vi "Valid.vi"(11 "ObserverSet in":refnum<class "ObserverSet.lvclass">) -> (2 "Valid?":bool, 3 "ObserverSet out":refnum<class "ObserverSet.lvclass">)   [LabVIEW 2011, in "Messenging.lvlib" / "ObserverSet.lvclass"]
uses:
  ObserverSet.lvclass
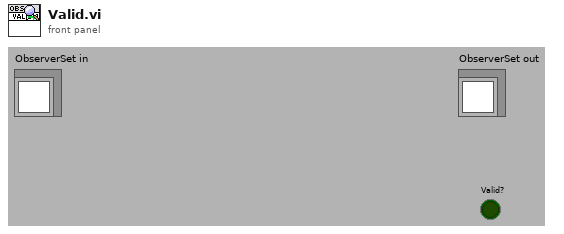
[diagram p1: front panel]
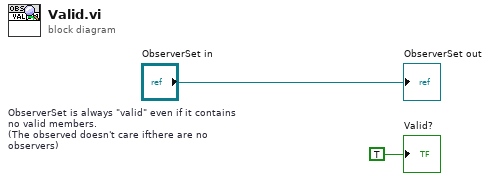
[diagram p0: block diagram]
diagram:
  w1 = TRUE  # ObserverSet is always "valid" even if it contains no valid members. (The observed doesn't care ifthere are no observers)
  "ObserverSet out" <- "ObserverSet in"
  "Valid?" <- w1
